vi "Import data from S2DS- Reader.vi"(8 "error in (no error)":errorcluster, 11 "connection id":refnum<k13>) -> (0 "error out":errorcluster, 2 "Data out":dbl[](array[numeric]), 3 "connection out":refnum<k13>)   [LabVIEW 2016]
doc: "Uses DataSocket to read array data. \n \nThe Writer, Server, and Reader can all be on the same computer or different computers. The Writer and Reader URLs should point to the computer where the DataSocket Server is."
panel:
  # "Overview: Demonstrates the use of the DataSocket functions to read data from the DataSocket server of S2DS.\nRequirements: Windows\nInstructions:\n1. Ensure Simple 2D Sweep : Export data  is TRUE.\n2. Run the VI."
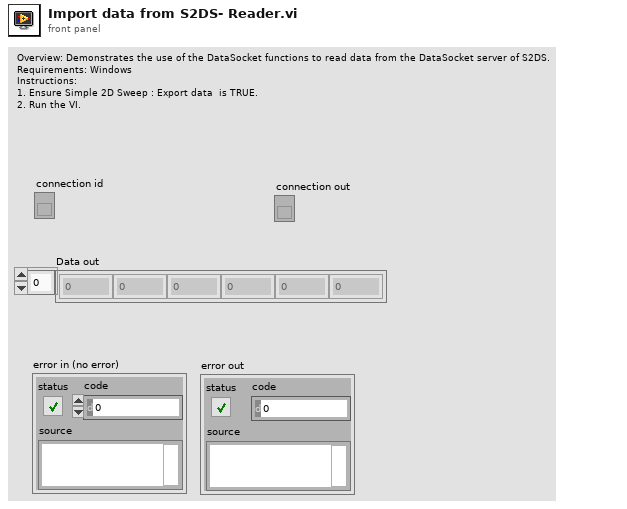
[diagram p1: front panel]
types:
  T1 = enum16{"Read", "Write", "ReadWrite", "BufferedRead", "BufferedReadWrite"}
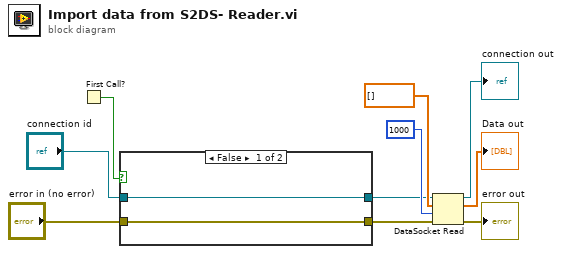
[diagram p0: block diagram]
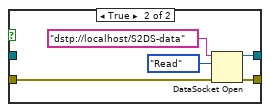
[diagram p2: hidden frame]
diagram:
  n1 = First Call?() -> (First Call?: T/F=w6:bool)
  n2 = case shown="False" w6 {
    tunnel: [w12 w15] -> w5
    tunnel: "connection id" -> [w12 _]
    tunnel: "error in (no error)" -> [w11 w14]
    tunnel: [w11 w13] -> w2
    frame False {
    }
    frame True {
      n3 = DataSocket Open(8:w14, 10:T1."Read" ("mode"), 11:"dstp://localhost/S2DS-data" ("Read Location")) -> (0:w13:errorcluster, 3:w15:refnum<k13>)  [unwired: 1 in]
    }
  }
  n4 = DataSocket Read(8:w2, 9:1000 ("ms timeout (10000)"), 10:dbl[] [], 11:w5) -> (0:→"error out":errorcluster, 2:→"Data out":dbl[], 3:→"connection out":refnum<k13>)  [unwired: 5 out]
